vi "Lidar Subsystem with Legit Chirp.vi"() -> ()   [LabVIEW 2009]
uses:
  <vilib>/rvi/FXPMathLib/FxpSinAndCos/XNode/nifxpmath_SinAndCos.xnode
  <vilib>/rvi/FXPMathLib/FxpAdd/XNode/nifxpmath_Add.xnode
  <vilib>/rvi/FXPMathLib/FxpAdd/simVIs/DllFxpAddTemp_sub.vi
  <vilib>/fxp/LVFixedPointOverflowPolicyTypeDef.ctl
  <vilib>/fxp/LVFixedPointQuantizationPolicyTypeDef.ctl
  <vilib>/rvi/FXPMathLib/FxpAdd/subVIs/nifxpmath_Add_SimConfig.ctl
  Motor Control Global.vi
  <vilib>/rvi/FXPMathLib/FxpMul/XNode/nifxpmath_Multiplier.xnode
  Test/Lidar Chirp Global.vi
  Motor Output Global.vi
  <vilib>/rvi/FXPMathLib/FxpMul/simVIs/DllFxpMulTemp_sub.vi
  <vilib>/rvi/FXPMathLib/FxpMul/subVIs/nifxpmath_Mul_SimConfig.ctl
  <vilib>/rvi/FXPMathLib/FxpSinAndCos/simVIs/DllFxpSinAndCosTemp_sub.vi
  <vilib>/rvi/FXPMathLib/FxpSinAndCos/subVIs/nifxpmath_SinAndCos_SimConfig.ctl
panel:
  in  "frequency, in pi rad Loop Frequency":fxp<+/-,16,1> format="%.16g"
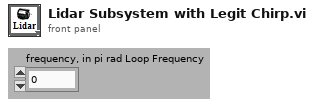
[diagram p1: front panel]
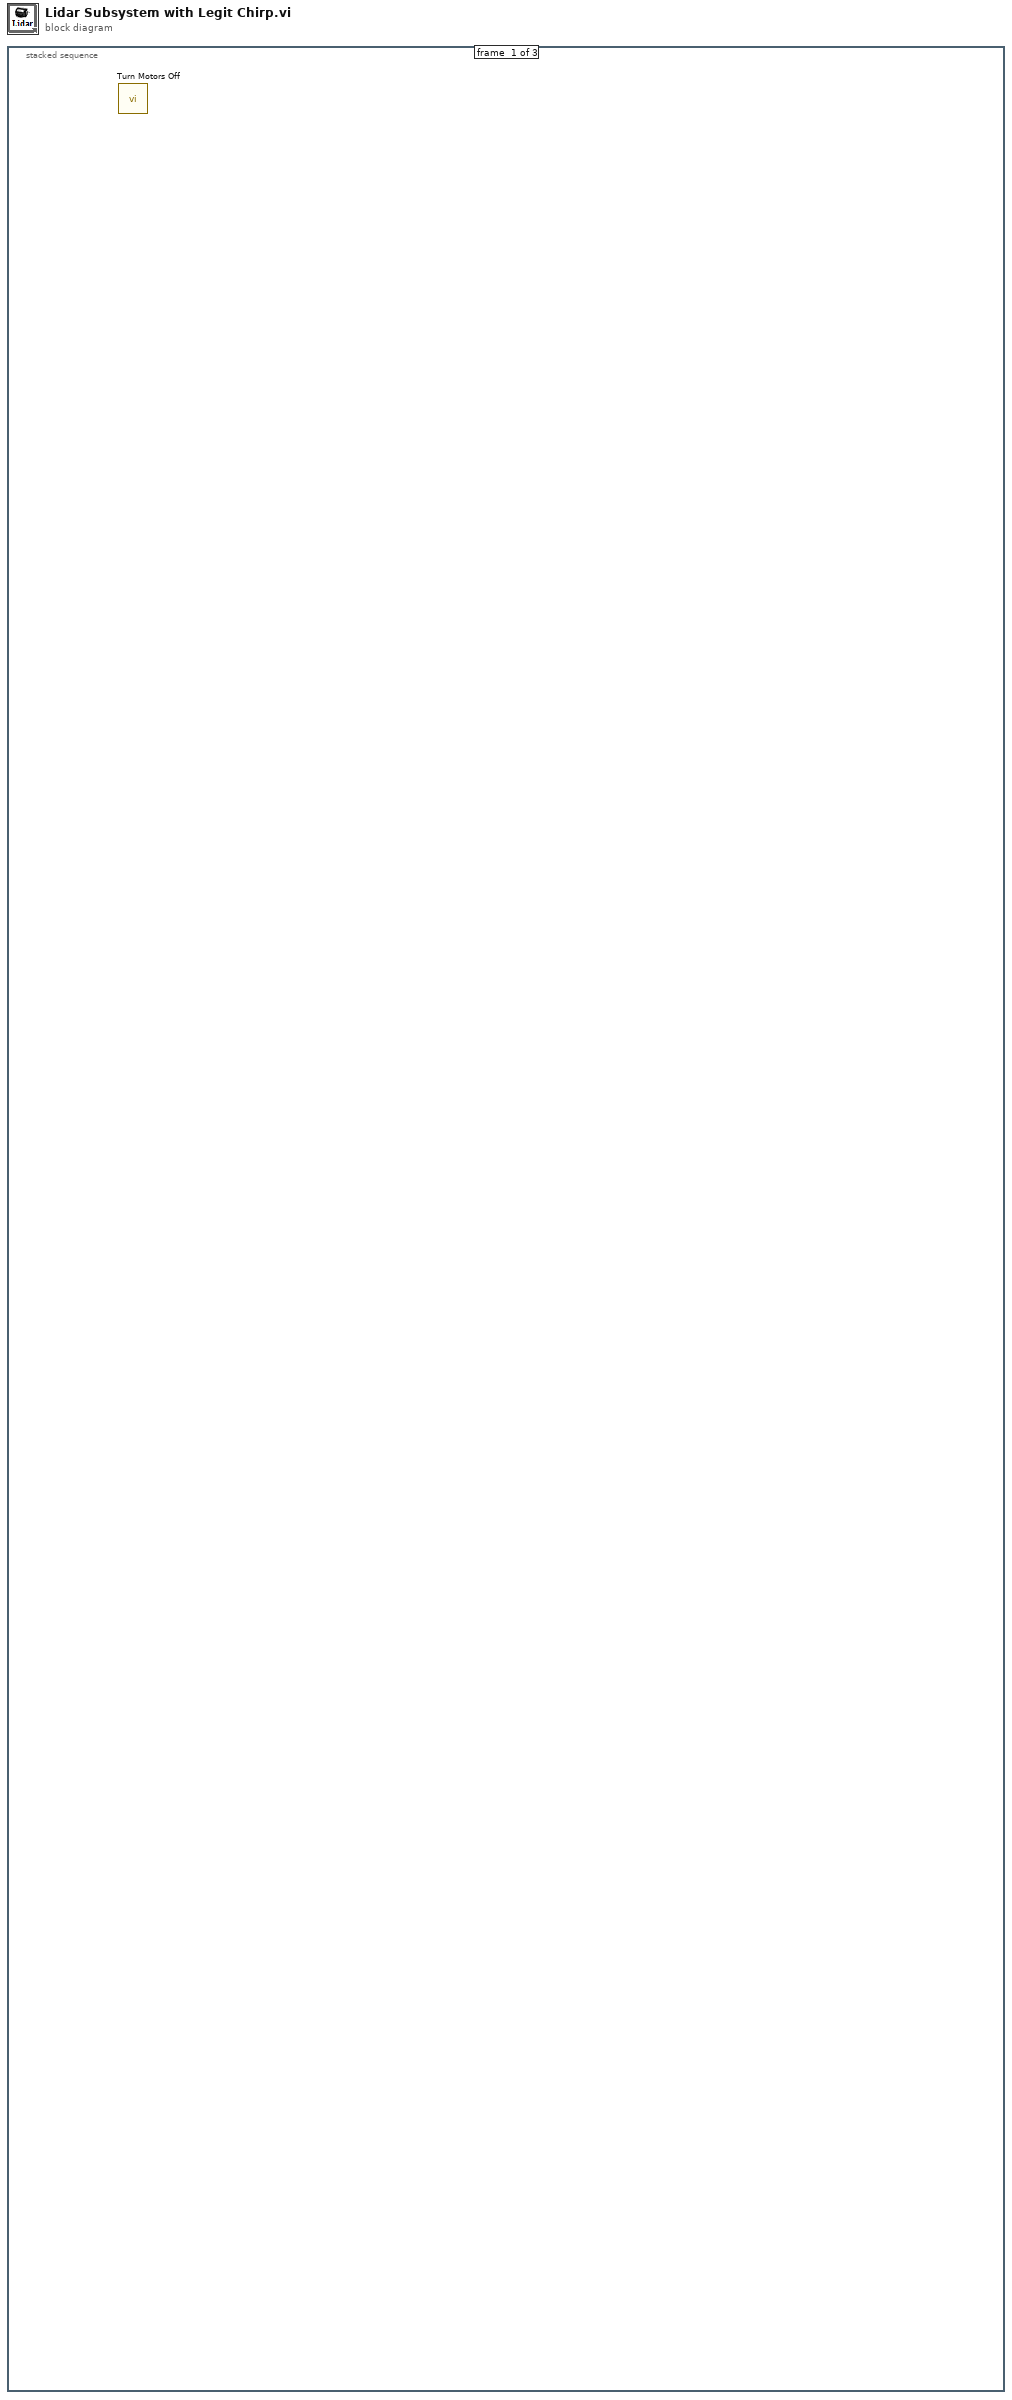
[diagram p0: block diagram]
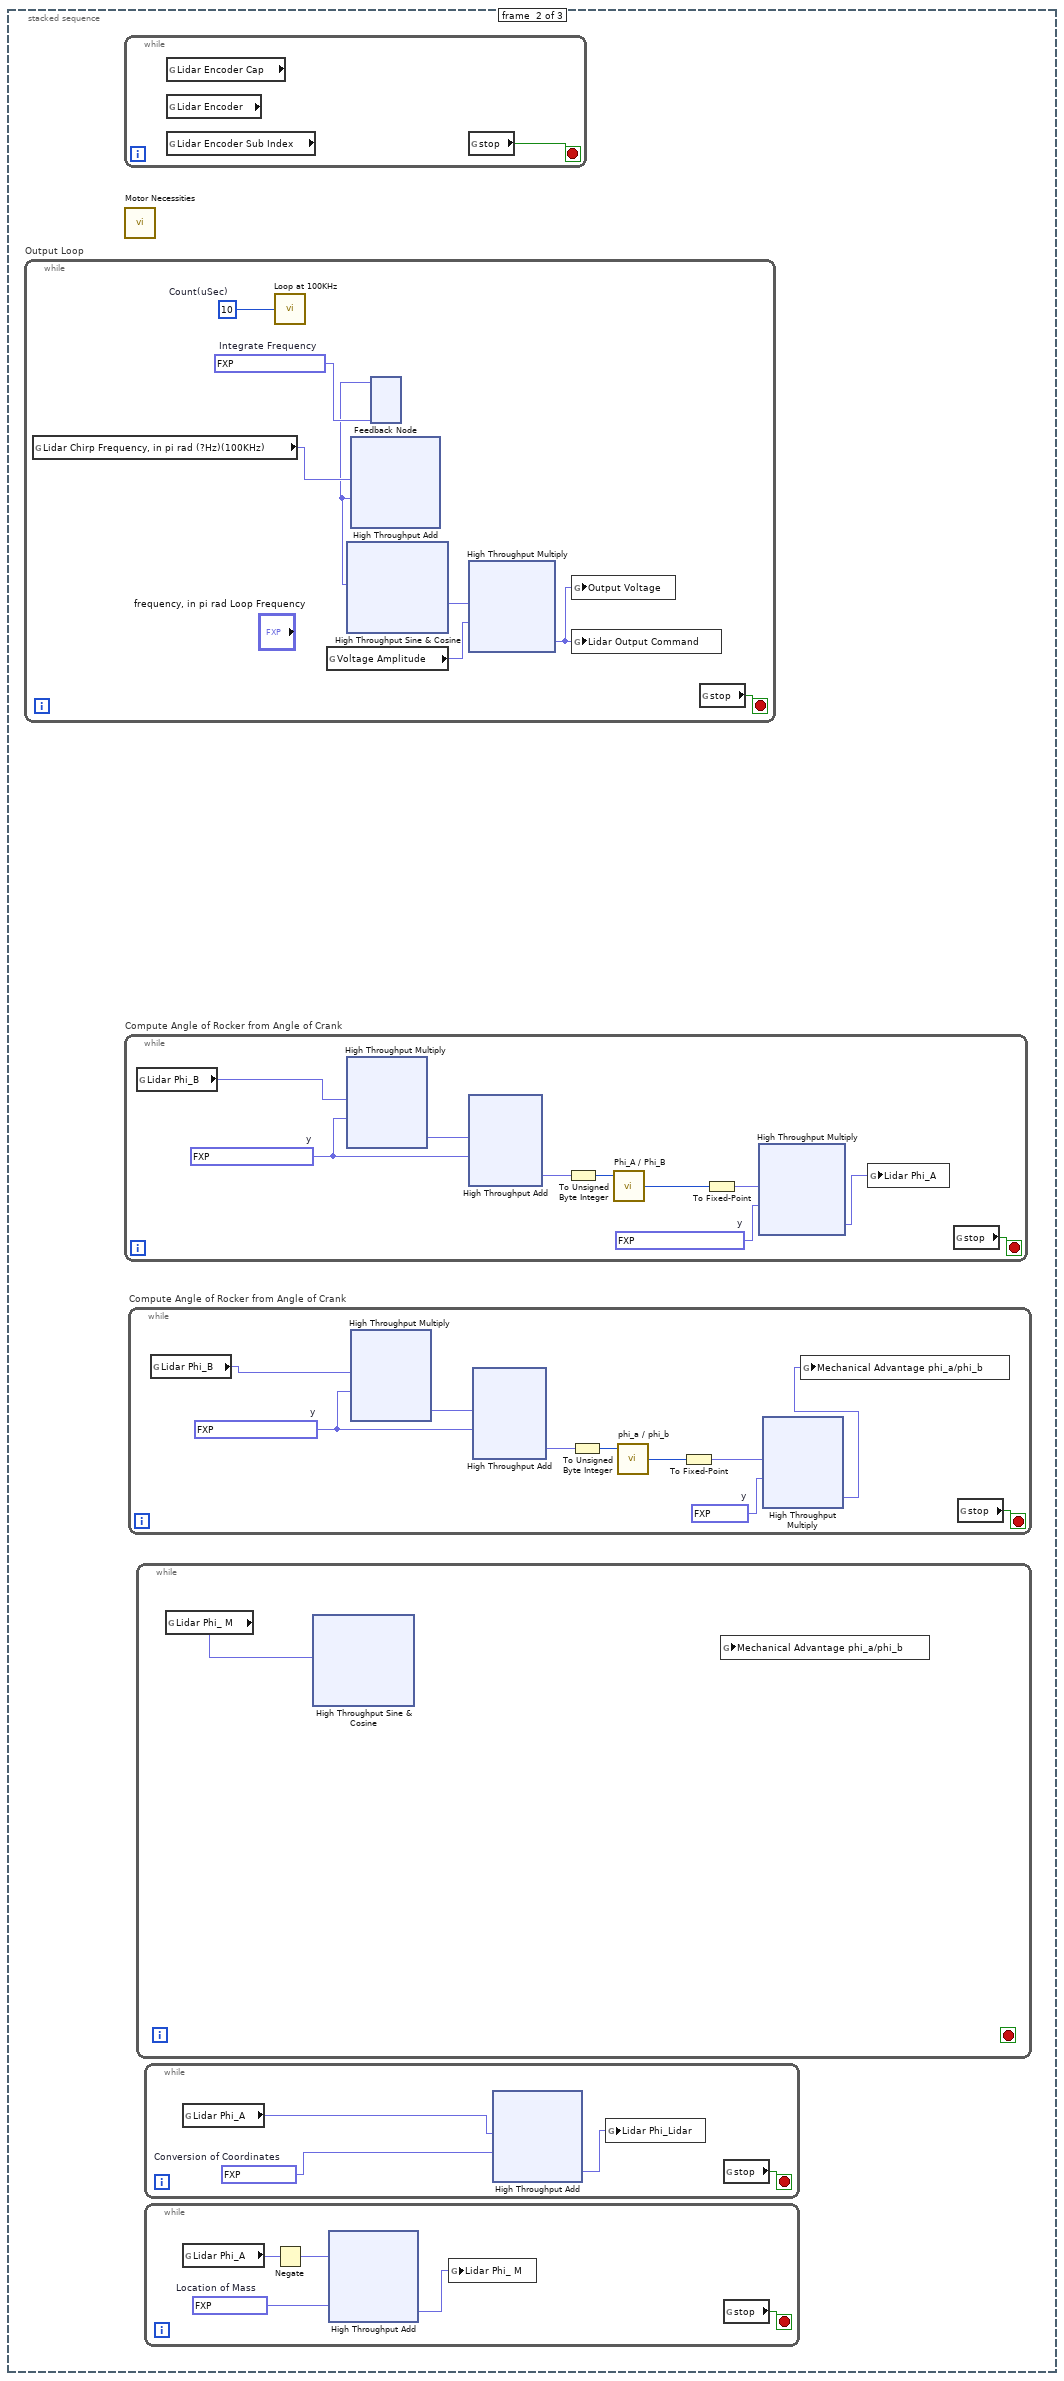
[diagram p2: hidden frame]
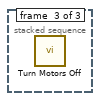
[diagram p3: hidden frame]
diagram:
  n1 = stacked-sequence {
    frame #0 {
      n2 = call "Turn Motors Off.vi"() -> ()  [unwired: 1 in]
    }
    frame #1 {
      n3 = while "Output Loop" {
        stop <- w288 stop-if-true
        w284 = u32 10  # Count(uSec)
        w289 = fxp<+/-,20,1> 0.0  # Integrate Frequency
        n4 = global read "Lidar Chirp Global.vi" "Lidar Chirp Frequency, in pi rad (?Hz)(100KHz)"() -> (w283:fxp<+/-,20,1>)
        n5 = call "Loop at 100KHz"("Count(uSec)"=w284) -> ()  [unwired: 1 out]
        n6 = global read "Lidar Chirp Global.vi" "Voltage Amplitude"() -> (w285:fxp<+/-,20,5>)
        n7 = feedback #1(w289) -> (w282:fxp<+/-,20,1>)
        n8 = xnode ("High Throughput Sine & Cosine")("x (pi)"=w282) -> ("sin(x)"=w287:fxp<+/-,16,2>)  [unwired: 1 out]
        n9 = xnode "High Throughput Add"("x"=w283, "y"=w282) -> ("x+y"=w290:fxp<+/-,20,1>)
        n10 = xnode "High Throughput Multiply"("x"=w287, "y"=w285) -> ("x*y"=w286:fxp<+/-,20,5>)
        n11 = global write "Lidar Chirp Global.vi" "Output Voltage"(w286) -> ()
        n12 = global write "Motor Output Global.vi" "Lidar Output Command"(w286) -> ()
        n13 = global read "Motor Control Global.vi" "stop"() -> (w288:bool)
      }
      n14 = while {
        stop <- w281 stop-if-true
        n15 = global read "Motor Control Global.vi" "Lidar Encoder Cap"() -> ()  [unwired: 1 out]
        n16 = global read "Motor Control Global.vi" "Lidar Encoder"() -> ()  [unwired: 1 out]
        n17 = global read "Motor Control Global.vi" "Lidar Encoder Sub Index"() -> ()  [unwired: 1 out]
        n18 = global read "Motor Control Global.vi" "stop"() -> (w281:bool)
      }
      n19 = call "Motor Necessities.vi"() -> ()  [unwired: 1 in]
      n20 = while "Compute Angle of Rocker from Angle of Crank" {
        stop <- w190 stop-if-true
        w193 = fxp<+,8,8> 128.0  # y
        w195 = fxp<+/-,16,-3> 0.0026035308837890625  # y
        n21 = global read "Lidar Chirp Global.vi" "Lidar Phi_B"() -> (w188:fxp<+/-,10,1>)
        n22 = xnode "High Throughput Multiply"("x"=w188, "y"=w193) -> ("x*y"=w194:fxp<+/-,8,8>)
        n23 = xnode "High Throughput Add"("x"=w194, "y"=w193) -> ("x+y"=w192:fxp<+,8,8>)
        n24 = To Unsigned Byte Integer(number=w192) -> (unsigned 8bit integer=w191:u8)
        n25 = call "Phi_A / Phi_B"("address"=w191) -> ("data out"=w197:i8)  [unwired: 8 in]
        n26 = To Fixed-Point(number=w197) -> (fixed-point=w196:fxp<+/-,8,8>)  [unwired: 1 in]
        n27 = xnode "High Throughput Multiply"("x"=w196, "y"=w195) -> ("x*y"=w189:fxp<+/-,10,1>)
        n28 = global write "Lidar Chirp Global.vi" "Lidar Phi_A"(w189) -> ()
        n29 = global read "Motor Control Global.vi" "stop"() -> (w190:bool)
      }
      n30 = while "Compute Angle of Rocker from Angle of Crank" {
        stop <- w66 stop-if-true
        w69 = fxp<+,8,8> 128.0  # y
        w71 = fxp<+,1,-6> 0.0078125  # y
        n31 = global read "Lidar Chirp Global.vi" "Lidar Phi_B"() -> (w64:fxp<+/-,10,1>)
        n32 = xnode "High Throughput Multiply"("x"=w64, "y"=w69) -> ("x*y"=w70:fxp<+/-,8,8>)
        n33 = xnode "High Throughput Add"("x"=w70, "y"=w69) -> ("x+y"=w68:fxp<+,8,8>)
        n34 = To Unsigned Byte Integer(number=w68) -> (unsigned 8bit integer=w67:u8)
        n35 = call "phi_a / phi_b"("address"=w67) -> ("data out"=w73:i8)  [unwired: 8 in]
        n36 = To Fixed-Point(number=w73) -> (fixed-point=w72:fxp<+/-,8,8>)  [unwired: 1 in]
        n37 = xnode "High Throughput Multiply"("x"=w72, "y"=w71) -> ("x*y"=w65:fxp<+/-,8,1>)
        n38 = global write "Lidar Chirp Global.vi" "Mechanical Advantage phi_a/phi_b"(w65) -> ()
        n39 = global read "Motor Control Global.vi" "stop"() -> (w66:bool)
      }
      n40 = while {
        stop <- _ stop-if-true
        n41 = global read "Lidar Chirp Global.vi" "Lidar Phi_ M"() -> (w33:fxp<+/-,10,1>)
        n42 = xnode "High Throughput Sine & Cosine"("x (pi)"=w33) -> ()  [unwired: 2 out]
        n43 = global read "Lidar Chirp Global.vi" "Mechanical Advantage phi_a/phi_b"() -> ()  [unwired: 1 in]
      }
      n44 = while {
        stop <- w160 stop-if-true
        w157 = fxp<+/-,10,1> 0.103515625  # Conversion of Coordinates
        n45 = global read "Lidar Chirp Global.vi" "Lidar Phi_A"() -> (w159:fxp<+/-,10,1>)
        n46 = xnode "High Throughput Add"("x"=w159, "y"=w157) -> ("x+y"=w158:fxp<+/-,10,1>)
        n47 = global write "Lidar Chirp Global.vi" "Lidar Phi_Lidar"(w158) -> ()
        n48 = global read "Motor Control Global.vi" "stop"() -> (w160:bool)
      }
      n49 = while {
        stop <- w5 stop-if-true
        w2 = fxp<+/-,10,1> 0.3046875  # Location of Mass
        n50 = global read "Lidar Chirp Global.vi" "Lidar Phi_A"() -> (w4:fxp<+/-,10,1>)
        n51 = Negate(x=w4) -> (-x=w1:fxp<+/-,11,2>)
        n52 = xnode "High Throughput Add"("x"=w1, "y"=w2) -> ("x+y"=w3:fxp<+/-,10,1>)
        n53 = global write "Lidar Chirp Global.vi" "Lidar Phi_ M"(w3) -> ()
        n54 = global read "Motor Control Global.vi" "stop"() -> (w5:bool)
      }
    }
    frame #2 {
      n55 = call "Turn Motors Off.vi"() -> ()  [unwired: 1 in]
    }
  }
